vi "波形存储(子VI).vi"(11 "ORP滴定曲线":u16[](graph)) -> ()   [LabVIEW 2016, in "斯坦道CODMn.lvlib"]
uses:
  <vilib>/Utility/sysdir.llb/System Directory Type.ctl
  <vilib>/Waveform/WDTFileIO.llb/ Write Waveform to File.vi
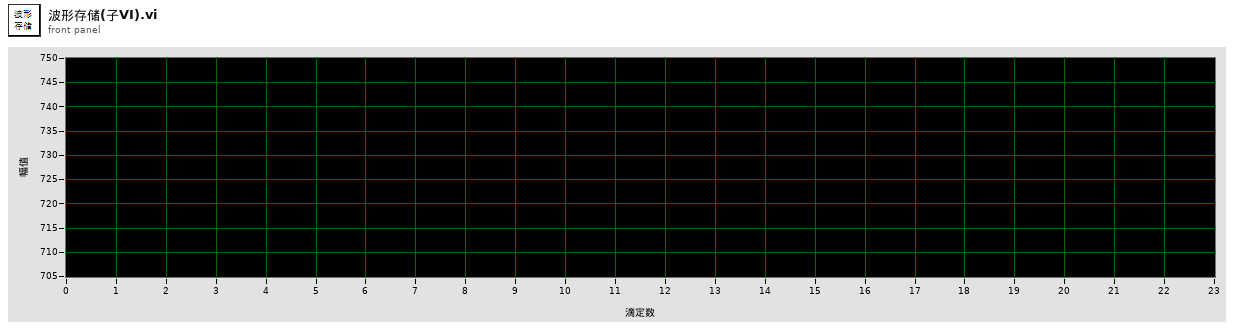
[diagram p1: front panel]
types:
  T1 = typedef "System Directory Type.ctl" = i32
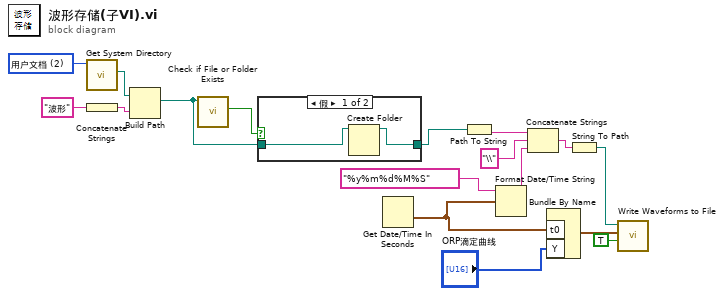
[diagram p0: block diagram]
diagram:
  w4 = T1 2 items=["用户目录"=0, "用户桌面"=1, "用户文档"=2, "用户应用程序数据"=3, "用户设置"=4, "用户临时目录"=5, "公共文档"=6, "公共应用程序数据"=7, "公共设置"=8, "公共缓存"=13, "系统核心库"=9, "系统安装库"=10, "应用程序文件"=11, "启动盘根目录"=12] ("system directory type")
  n1 = call <vilib>:"Get System Directory.vi"("system directory type"=w4) -> ("system directory"=w3:path)  [unwired: 10 in]
  n2 = Concatenate Strings("波形" ("condition")) -> (w1:string)
  n3 = Build Path(base path=w3, name or relative path=w1) -> (appended path=w6:path)
  n4 = call <vilib>:"Check if File or Folder Exists.vi"("path"=w6) -> ("file or folder exists?"=w5:bool)  [unwired: 8 in, 2 out]
  n5 = case shown="假" w5 {
    tunnel: w6 -> [w19 w20]
    tunnel: [w18 w20] -> w16
    frame False {
      n6 = Create Folder(path (use dialog)=w19) -> (created path=w18:path)  [unwired: 2 in, 2 out]
    }
    frame True {
    }
  }
  n7 = Get Date/Time In Seconds() -> (seconds since 1Jan1904=w12:timestamp)
  n8 = Path To String(path=w16) -> (string=w8:string)
  n9 = Format Date/Time String(time format string (%c)="%y%m%d%M%S" ("时间格式字符串(%c)"), seconds (now)=w12) -> (date/time string=w14:string)  [unwired: 1 in]
  n10 = Concatenate Strings(w8, "\\" ("字符串"), w14) -> (w10:string)
  n11 = Bundle By Name("t0"=w12, "Y"="ORP滴定曲线") -> (w7:waveform(u16))  [unwired: 1 in]
  n12 = String To Path(string=w10) -> (path=w11:path)
  n13 = call-poly <vilib>:"Write Waveforms to File.vi"("append to file? (new file:F)"=TRUE, "waveform"=w7, "file path (dialog if empty)"=w11) -> ()  [unwired: 7 in, 2 out]
